vi "CRYView Pic WAIT Curver.vi"(9 "sData":string="BRIDGE_OUT", 11 "cView":T1) -> (3 "cView_Out":T1)   [LabVIEW 2013]
uses:
  CRYView Global.vi
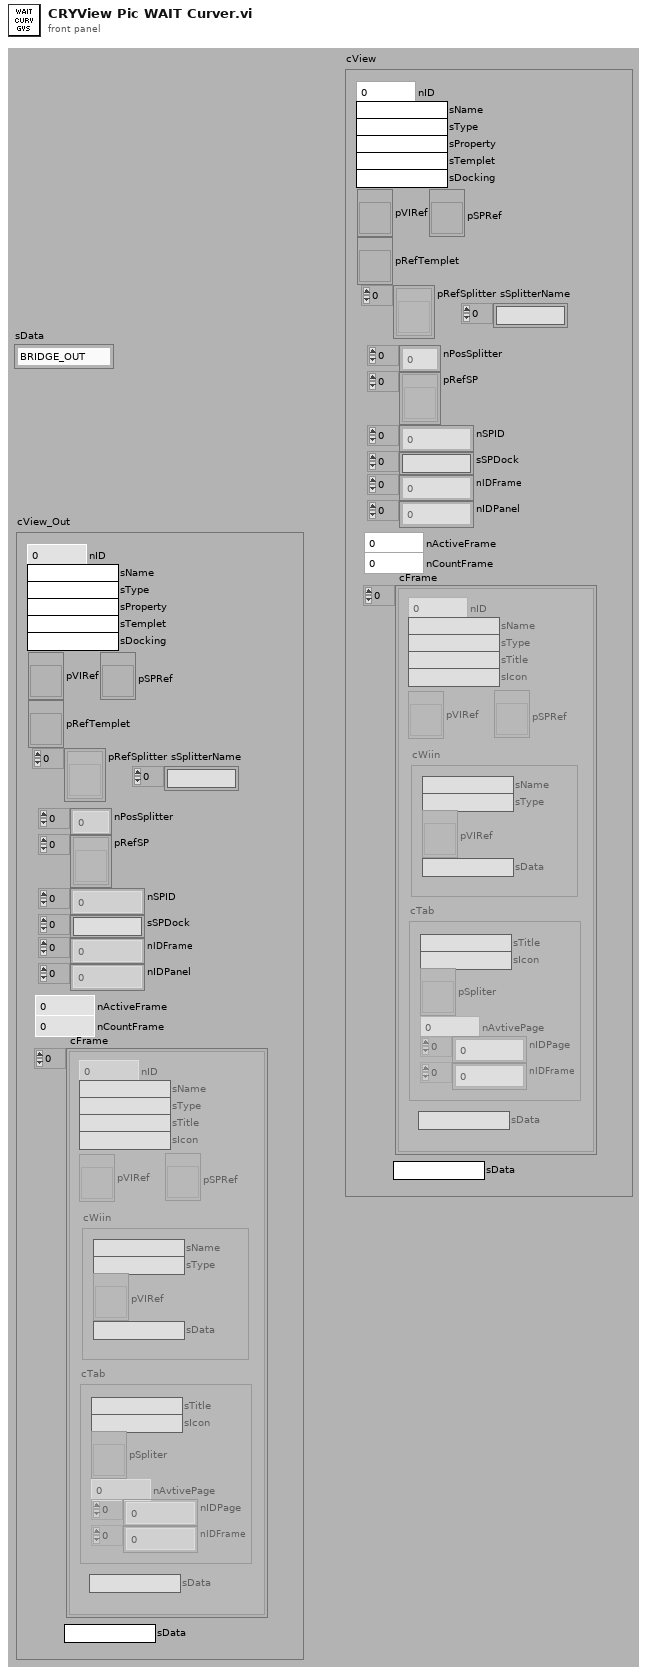
[diagram p1: front panel]
types:
  T1 = cluster{"nID":i32, "sName":string, "sType":string, "sProperty":string, "sTemplet":string, "sDocking":string, "pVIRef":refnum<vi>, "pSPRef":refnum<vi>, "pRefTemplet":refnum<vi>, "pRefSplitter":refnum<vi>[], "nPosSplitter":i32[], "pRefSP":refnum<vi>[], "nSPID":i32[], "sSPDock":string[], "nIDFrame":i32[], "nIDPanel":i32[], "nActiveFrame":i32, "nCountFrame":i32, "cFrame":cluster{"nID":i32, "sName":string, "sType":string, "sTitle":string, "sIcon":string, "pVIRef":refnum<vi>, "pSPRef":refnum<vi>, "cWiin":cluster{"sName":string, "sType":string, "pVIRef":refnum<vi>, "sData":string}, "cTab":cluster{"sTitle":string, "sIcon":string, "pSpliter":refnum<vi>, "nAvtivePage":i32, "nIDPage":i32[], "nIDFrame":i32[]}, "sData":string}[], "sData":string, "sSplitterName":string[]}
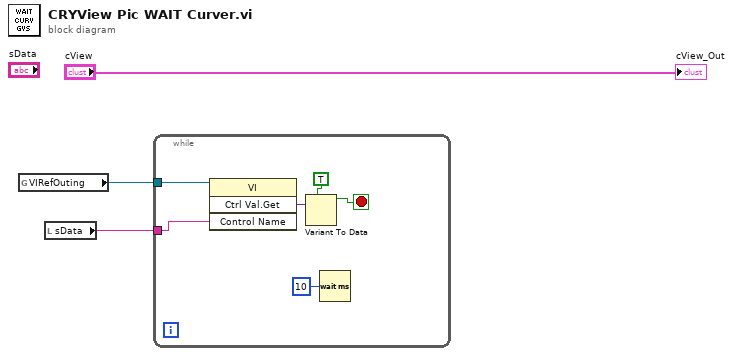
[diagram p0: block diagram]
diagram:
  n1 = global read "CRYView Global.vi" "VIRefOuting"() -> (w3:refnum<vi>)
  n2 = local read "sData"() -> (w2:string)
  n3 = while {
    tunnel: w3 -> [w9]
    tunnel: w2 -> [w8]
    stop <- w5 stop-if-true
    n4 = invoke class="VI" method="Ctrl Val.Get"(reference=w9, "Control Name"=w8) -> ("Get Control Value Variant"=w7:variant)  [unwired: 2 in, 3 out]
    n5 = Variant To Data(type=TRUE, Variant=w7) -> (data=w5:bool)  [unwired: 1 in, 1 out]
    n6 = Wait (ms)(milliseconds to wait=u32 10) -> ()  [unwired: 1 out]
  }
  "cView_Out" <- "cView"
